vi "PF_ModifyExtrema.vi"(8 "Max Voltage Range?":bool, 9 "Extremas Array In":T1(array[cluster]), 11 "Intensity Array":dbl[](array[numeric])) -> (1 "Extremas Array Out":T1(array[cluster]))   [LabVIEW 2020]
panel:
  # "Phase Fitter: Modify Extrema"
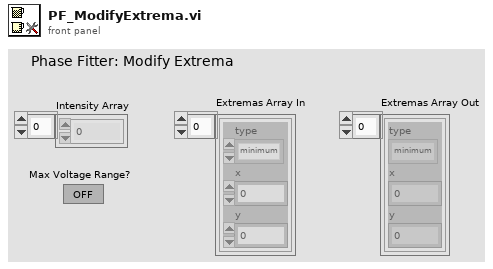
[diagram p1: front panel]
types:
  T1 = cluster{"type":enum16{"minimum", "maximum"}, "x":i32, "y":dbl}[]
  T2 = cluster{"type":enum16{"minimum", "maximum"}, "x":i32, "y":dbl}
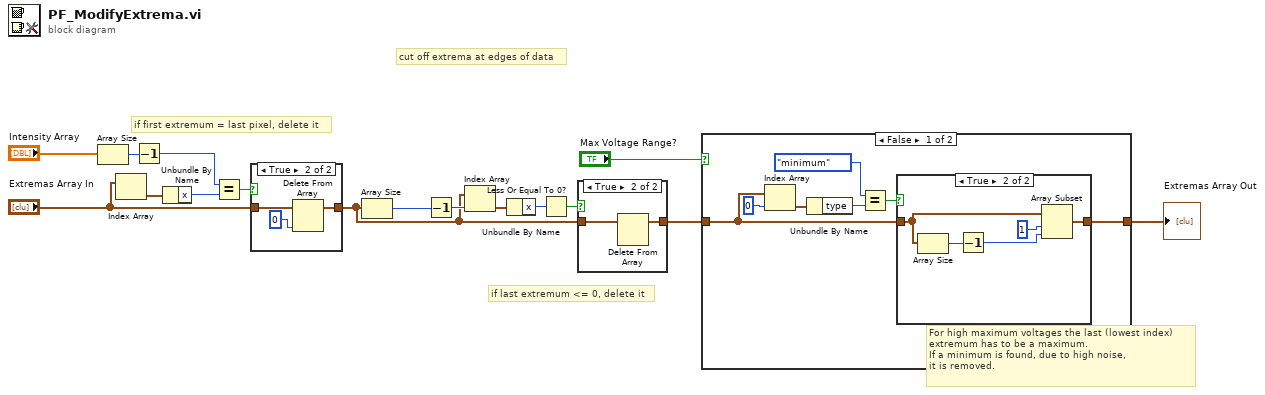
[diagram p0: block diagram]
diagram:
  # "if last extremum <= 0, delete it"
  # "if first extremum = last pixel, delete it"
  # "cut off extrema at edges of data"
  n1 = Array Size(array="Intensity Array") -> (size(s)=w5:i32)
  n2 = Index Array(array="Extremas Array In") -> (element=w8:T2)  [unwired: 1 in]
  n3 = Decrement(x=w5) -> (x-1=w7:i32)
  n4 = Unbundle By Name(w8) -> ("x"=w9:i32)
  n5 = Equal?(x=w7, y=w9) -> (x = y?=w12:bool)
  n6 = case shown="True" w12 {
    tunnel: [w17 w19] -> w13
    tunnel: "Extremas Array In" -> [w17 w20]
    frame False {
    }
    frame True {
      n7 = Delete From Array(array=w20, index=0) -> (array with subset deleted=w19:T1)  [unwired: 1 in, 1 out]
    }
  }
  n8 = Array Size(array=w13) -> (size(s)=w6:i32)
  n9 = Decrement(x=w6) -> (x-1=w16:i32)
  n10 = Index Array(array=w13, index=w16) -> (element=w10:T2)
  n11 = Unbundle By Name(w10) -> ("x"=w11:i32)
  n12 = Less Or Equal To 0?(x=w11) -> (x <= 0?=w15:bool)
  n13 = case shown="True" w15 {
    tunnel: [w21 w22] -> w14
    tunnel: w13 -> [w21 w23]
    frame False {
    }
    frame True {
      n14 = Delete From Array(array=w23) -> (array with subset deleted=w22:T1)  [unwired: 2 in, 1 out]
    }
  }
  n15 = case shown="False" "Max Voltage Range?" {
    tunnel: [w30 w37] -> w1
    tunnel: w14 -> [w29 w37]
    frame False {
      # "For high maximum voltages the last (lowest index)\nextremum has to be a maximum.\nIf a minimum is found, due to high noise,\nit is removed."
      n16 = Index Array(array=w29, index=0 ("Index")) -> (element=w24:T2)
      n17 = Unbundle By Name(w24) -> ("type"=w26:enum16{"minimum", "maximum"})
      n18 = Equal?(x=enum16{"minimum", "maximum"}."minimum" ("Output Element"), y=w26) -> (x = y?=w28:bool)
      n19 = case shown="True" w28 {
        tunnel: w29 -> [w31 w32]
        tunnel: [w31 w35] -> w30
        frame False {
        }
        frame True {
          n20 = Array Size(array=w32) -> (size(s)=w34:i32)
          n21 = Decrement(x=w34) -> (x-1=w33:i32)
          n22 = Array Subset(array=w32, index=1 ("Array Index"), length=w33) -> (w35:T1)
        }
      }
    }
    frame True {
      # "for low voltages the first extremum\ncan be an maximum"
    }
  }
  "Extremas Array Out" <- w1
